vi "sub_9215-main.vi"(8 "error in":errorcluster) -> (0 "error out":errorcluster)   [LabVIEW 2013]
uses:
  Global.vi
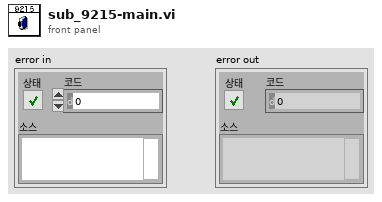
[diagram p1: front panel]
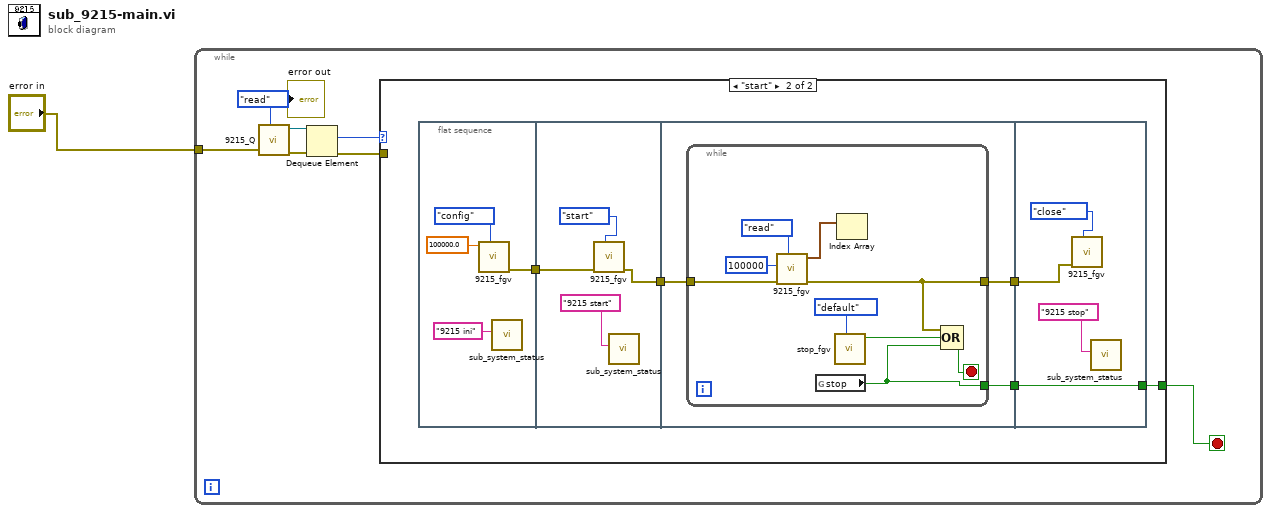
[diagram p0: block diagram]
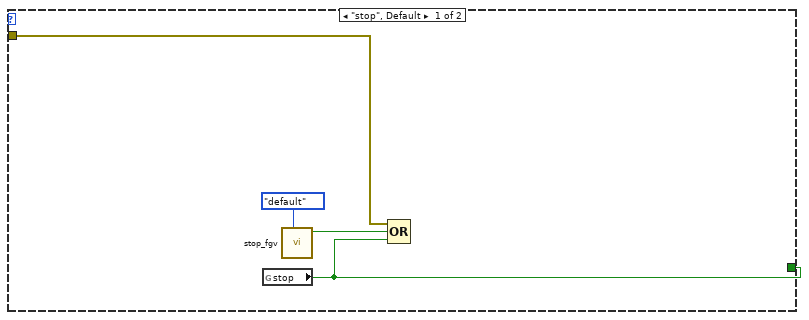
[diagram p2: hidden frame]
diagram:
  n1 = while {
    tunnel: "error in" -> [w8]
    stop <- w2 stop-if-true
    n2 = call "9215_Q.vi"("cmd"=enum16{"close", "write", "read", "create"}."read", "error in"=w8) -> ("error out"=w6:errorcluster, "queue out"=w5:refnum<queue>)  [unwired: 8 in]
    n3 = Dequeue Element(queue=w5, error in (no error)=w6) -> (element=w4:enum16{"stop", "start"}, error out=w3:errorcluster)  [unwired: 1 in, 2 out]
    n4 = case shown="\"start\"" w4 {
      tunnel: w3 -> [w10 _]
      tunnel: [w9 w14] -> w2
      frame "stop", Default {
        n5 = global read "Global.vi" "stop"() -> (w9:bool)
        n6 = call "stop_fgv.vi"("cmd"=enum16{"default", "ini", "stop"}."default") -> ("stop"=w11:bool)  [unwired: 9 in, 1 out]
        n7 = Compound Arithmetic op=OR(w10, w11, w9) -> ()  [unwired: 1 out]
      }
      frame "start" {
        n8 = flat-sequence {
          tunnel: [w19] -> w17
          tunnel: w17 -> [w24]
          tunnel: [w23] -> w16
          tunnel: w16 -> [w28]
          tunnel: [w27] -> w15
          tunnel: [w26] -> w13
          tunnel: w15 -> [w40]
          tunnel: [w38] -> w14
          tunnel: w13 -> [w38]
          frame #0 {
            n9 = call "9215_fgv.vi"("cmd"=enum16{"config", "start", "read", "close"}."config", "rate"=100000.0) -> ("error out"=w19:errorcluster)  [unwired: 8 in, 1 out]
            n10 = call "sub_system_status.vi"("String in"="9215 ini") -> ()  [unwired: 10 in, 1 out]
          }
          frame #1 {
            n11 = call "9215_fgv.vi"("cmd"=enum16{"config", "start", "read", "close"}."start", "error in"=w24) -> ("error out"=w23:errorcluster)  [unwired: 8 in, 1 out]
            n12 = call "sub_system_status.vi"("String in"="9215 start") -> ()  [unwired: 10 in, 1 out]
          }
          frame #2 {
            n13 = while {
              tunnel: w28 -> [w35]
              tunnel: [w30] -> w27
              tunnel: [w29] -> w26
              stop <- w31 stop-if-true
              n14 = call "9215_fgv.vi"("cmd"=enum16{"config", "start", "read", "close"}."read", "error in"=w35, "number of samples per channel"=100000) -> ("error out"=w30:errorcluster, "data"=w34:waveform(dbl)[])  [unwired: 7 in]
              n15 = global read "Global.vi" "stop"() -> (w29:bool)
              n16 = call "stop_fgv.vi"("cmd"=enum16{"default", "ini", "stop"}."default") -> ("stop"=w32:bool)  [unwired: 9 in, 1 out]
              n17 = Index Array(array=w34) -> ()  [unwired: 1 in, 1 out]
              n18 = Compound Arithmetic op=OR(w30, w32, w29) -> (w31:bool)
            }
          }
          frame #3 {
            n19 = call "9215_fgv.vi"("cmd"=enum16{"config", "start", "read", "close"}."close", "error in"=w40) -> ()  [unwired: 8 in, 2 out]
            n20 = call "sub_system_status.vi"("String in"="9215 stop") -> ()  [unwired: 10 in, 1 out]
          }
        }
      }
    }
  }
